vi "UpdateLimsTestStepValues.vi"(7 "step-id":u32, 8 "error in (no error)":errorcluster, 9 "duration hours":dbl, 10 "value":dbl, 11 "ByteQXAPIBase in":refnum<class "ByteQXAPIBase.lvclass">) -> (0 "error out":errorcluster, 2 "step result":T1, 3 "ByteQXAPIBase out":refnum<class "ByteQXAPIBase.lvclass">)   [LabVIEW 2019, in "ByteQXWebAPI.lvlib" / "ByteQXAPIBase.lvclass"]
doc: "Upload value and duration for a step and it returns the outcome"
uses:
  ByteQXAPIBase.lvclass
  TypeDef/UpdateLimsTestStepData.ctl
  Private/module.ctl
  ByteQXAPIBase.lvclass/ByteQXAPIBase.ctl
  <vilib>/Bytelabs/ByteREST/ByteRESTClass/ByteRESTBase/RESTBase.lvclass
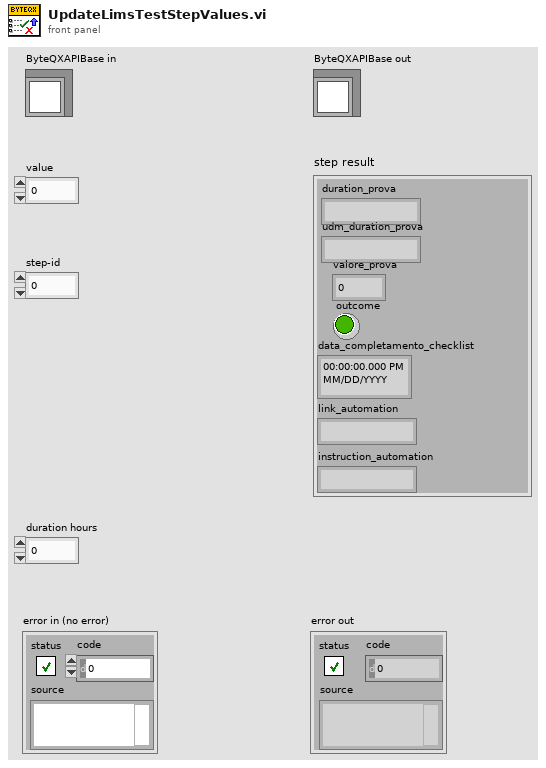
[diagram p1: front panel]
types:
  T1 = typedef "ByteQXWebAPI.lvlib/ByteQXAPIBase.lvclass/UpdateLimsTestStepData.ctl" = cluster{"outcome":bool, "data_completamento_checklist":timestamp, "udm_duration_prova":string, "valore_prova":dbl, "link_automation":string, "instruction_automation":string, "duration_prova":string}
  T2 = typedef "ByteQXWebAPI.lvlib/ByteQXAPIBase.lvclass/module.ctl" = enum16{"gs", "tms"}
  T3 = cluster{"duration_prova":string, "udm_duration_prova":string, "data_completamento_checklist":string, "valore_prova":dbl, "outcome":string, "link_automation":string, "instruction_automation":string}
  T4 = typedef "ByteQXWebAPI.lvlib/ByteQXAPIBase.lvclass/Step.ctl" = cluster{"id":i32, "descrizione":string, "prova":cluster{"slug":string}, "assets":T5[], "criterio_accettazione":string, "valore_criterio_accettazione_max":dbl, "valore_criterio_accettazione_min":dbl, "udm_criterio_accettazione":string, "duration_prova":string, "udm_duration_prova":string, "valore_prova":dbl, "ordine":i32, "user":i32, "link_automation":string, "instruction_automation":string, "data_completamento_checklist":timestamp, "outcome":bool, "step_type":string, "channels":string[]}
  T5 = typedef "ByteQXWebAPI.lvlib/ByteQXAPIBase.lvclass/Asset.ctl" = cluster{"descrizione":string, "slug":string, "id":i32}
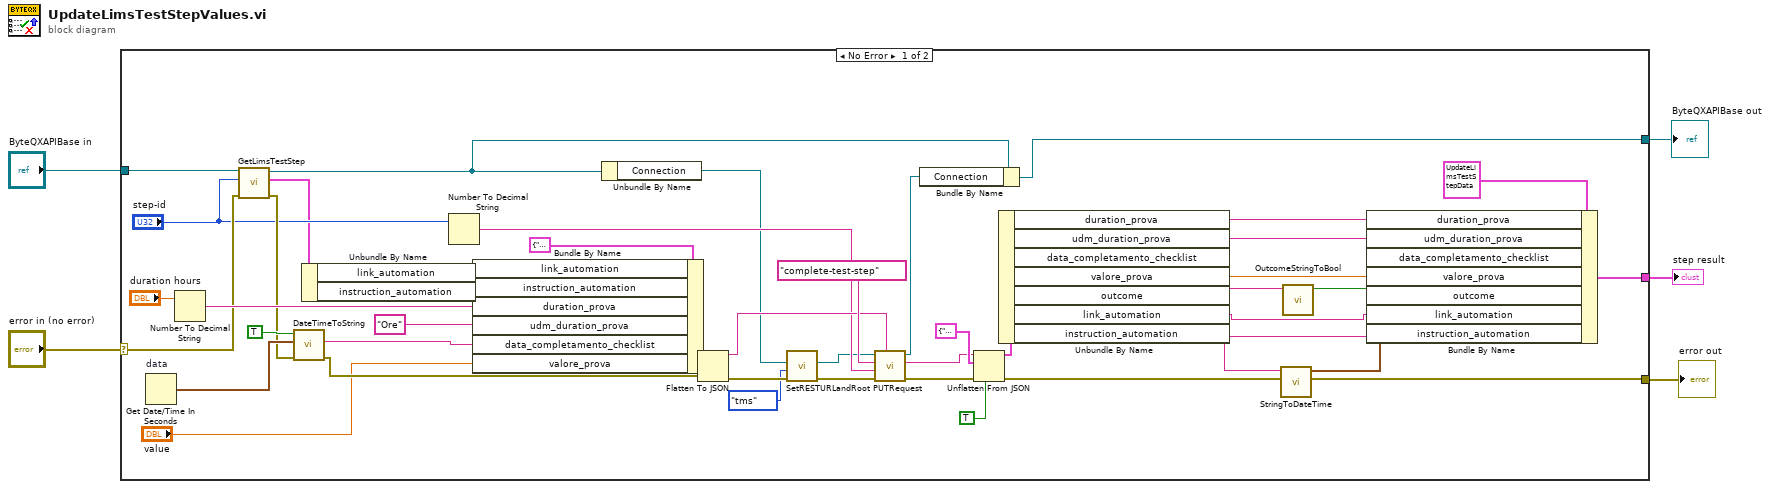
[diagram p0: block diagram]
diagram:
  n1 = case shown="No Error" "error in (no error)" {
    selector: "error in (no error)" -> [w21 w53]
    tunnel: [w30 w53] -> w4
    tunnel: [w51 w52] -> w2
    tunnel: "ByteQXAPIBase in" -> [w23 w52]
    tunnel: [w31 _] -> w1
    frame No Error {
      n2 = Get Date/Time In Seconds "data"() -> (seconds since 1Jan1904=w25:timestamp)
      n3 = Number To Decimal String(number="duration hours") -> (decimal integer string=w46:string)  [unwired: 1 in]
      n4 = call-dynamic "GetLimsTestStep.vi"("error in (no error)"=w21, "step-id"="step-id", "ByteQXAPIBase in"=w23) -> ("error out"=w20:errorcluster, "StepList"=w18:T4, "ByteQXAPIBase out"=w22:refnum<class "ByteQXAPIBase.lvclass">)  [unwired: 6 in]
      n5 = call "DateTimeToString.vi"("error in"=w20, "current time"=w25, "include Time?"=TRUE ("Time")) -> ("error out"=w43:errorcluster, "date string"=w44:string)  [unwired: 7 in]
      n6 = Unbundle By Name(w18) -> ("link_automation"=w17:string, "instruction_automation"=w16:string)
      n7 = Number To Decimal String(number="step-id") -> (decimal integer string=w28:string)  [unwired: 1 in]
      n8 = Bundle By Name(cluster=T3 {"duration_prova"="3", "udm_duration_prova"="Ore", "data_completamento_checklist"="2024-10-24T17:19:12Z", "valore_prova"=5.0, "outcome"="P", "link_automation"="", "instruction_automation"=""} ("Update Step"), "link_automation"=w17, "instruction_automation"=w16, "duration_prova"=w46, "udm_duration_prova"="Ore", "data_completamento_checklist"=w44, "valore_prova"="value") -> (w45:T3)
      n9 = Unbundle By Name(w22) -> ("Connection"=w7:refnum<class "RESTBase.lvclass">)
      n10 = Flatten To JSON(anything=w45, error in (no error)=w43) -> (JSON string=w48:string, 11:w10:errorcluster)  [unwired: 1 in]
      n11 = call "SetRESTURLandRoot.vi"("error in (no error)"=w10, "module"=module."tms", "ByteREST in"=w7) -> ("error out"=w9:errorcluster, "ByteREST out"=w8:refnum<class "RESTBase.lvclass">)  [unwired: 7 in]
      n12 = call-dynamic "PUTRequest.vi"("Body in"=w48, "error in (no error)"=w9, "Parameter"=w28, "Request"="complete-test-step", "ByteRESTBase in"=w8) -> ("error out"=w33:errorcluster, "Body"=w32:string, "ByteRESTBase out"=w50:refnum<class "RESTBase.lvclass">)  [unwired: 3 in, 1 out]
      n13 = Bundle By Name(cluster=w22, "Connection"=w50) -> (w51:refnum<class "ByteQXAPIBase.lvclass">)
      n14 = Unflatten From JSON(JSON string=w32, type and defaults=T3 {"duration_prova"="", "udm_duration_prova"="", "data_completamento_checklist"="", "valore_prova"=0.0, "outcome"="P", "link_automation"="", "instruction_automation"=""}, default null elements? (F)=TRUE, error in (no error)=w33) -> (value=w40:T3, error out=w34:errorcluster)  [unwired: 3 in]
      n15 = Unbundle By Name(w40) -> ("duration_prova"=w39:string, "udm_duration_prova"=w38:string, "data_completamento_checklist"=w36:string, "valore_prova"=w37:dbl, "outcome"=w12:string, "link_automation"=w13:string, "instruction_automation"=w14:string)
      n16 = call "StringToDateTime.vi"("error in (no error)"=w34, "datetime string"=w36) -> ("error out"=w30:errorcluster, "timestamp"=w35:timestamp)  [unwired: 8 in]
      n17 = call "OutcomeStringToBool.vi"("outcome string"=w12) -> ("outcome bool"=w11:bool)  [unwired: 10 in]
      n18 = Bundle By Name(cluster=T1 {"outcome"=FALSE, "data_completamento_checklist"=timestamp(0 s since 1904-01-01), "udm_duration_prova"="", "valore_prova"=0.0, "link_automation"="", "instruction_automation"="", "duration_prova"=""} ("Result Step"), "duration_prova"=w39, "udm_duration_prova"=w38, "data_completamento_checklist"=w35, "valore_prova"=w37, "outcome"=w11, "link_automation"=w13, "instruction_automation"=w14) -> (w31:T1)
    }
    frame Error {
    }
  }
  "error out" <- w4
  "ByteQXAPIBase out" <- w2
  "step result" <- w1
